vi "Set LED.vi"   [LabVIEW 2013]
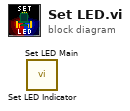
[diagram p0: block diagram]
diagram:
  n1 = call "Set LED Indicator.vi"() -> ()  [unwired: 1 in]
  n2 = call "Set LED Main.vi"() -> ()  [unwired: 1 in]
